vi "Initialization VI.vi"(8 "error in (no error)":errorcluster, 10 "Custom XML":string, 11 "Device Item Ref in":T1 format="%.0x") -> (0 "error out":errorcluster, 3 "Device Item Ref out":T1 format="%.0x")   [LabVIEW 2023, in "Vires VTD System Explorer.lvlib"]
uses:
  Vires VTD System Explorer.lvlib
  <vilib>/NI VeriStand/Custom Device API/Custom Device Item Ref.ctl
  Shared/Constants.vi
  <vilib>/NI VeriStand/Custom Device API/Custom Device API.lvlib
  Shared/Vires VTD Shared.lvlib
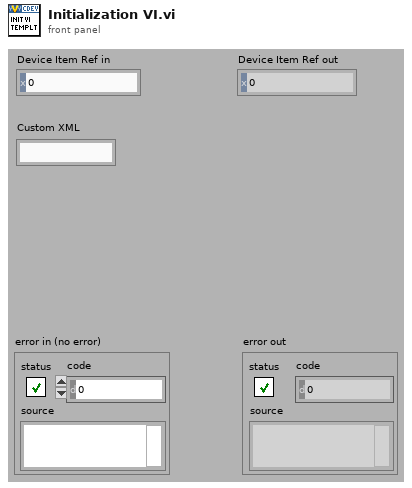
[diagram p1: front panel]
types:
  T1 = typedef "Custom Device API.lvlib/Custom Device Item Ref.ctl" = u64
  T2 = typedef "Vires VTD Shared.lvlib/Network Settings.ctl" = cluster{"IP adress":string, "RDB":cluster{"Protocol":T3, "Tx Port":u16, "Rx Port":u16, "Buffer Size":i32, "Timeout":u16}, "SCP":cluster{"Protocol":T3, "Tx Port":u16, "Rx Port":u16, "Buffer Size":i32, "Timeout":u16}}
  T3 = typedef "Vires VTD Shared.lvlib/Protocol.ctl" = enum16{"UDP", "TCP"}
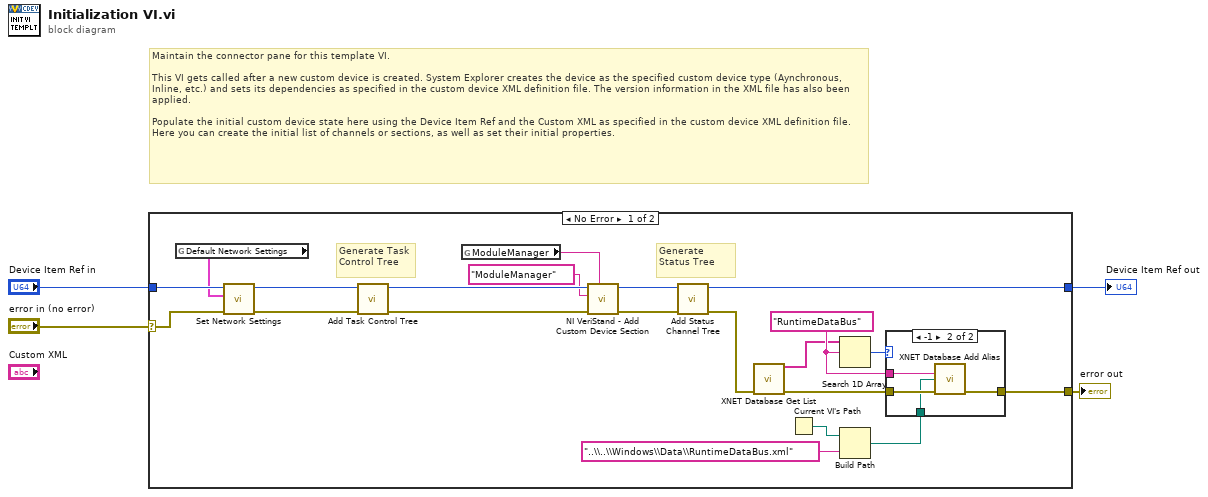
[diagram p0: block diagram]
diagram:
  # "Maintain the connector pane for this template VI.\n\nThis VI gets called after a new custom device is created. System Explorer creates the device as the specified custom device type (Aynchronous, Inline, etc.) and sets its dependencies as specified in the custom device XML definition file. The version information in the XML file has also been applied.\n\nPopulate the initial custom device state here using the Device Item Ref and the Custom XML as specified in the custom device XML definition file. Here you can create the initial list of channels or sections, as well as set their initial properties."
  n1 = case shown="No Error" "error in (no error)" {
    selector: "error in (no error)" -> [w13 w32]
    tunnel: [w17 w32] -> w1
    tunnel: [w19 w31] -> w3
    tunnel: "Device Item Ref in" -> [w15 w31]
    frame No Error {
      w23 = "RuntimeDataBus" ("element")
      # "Generate Status Tree"
      # "Generate Task Control Tree"
      n2 = global read "Constants.vi" "Default Network Settings"() -> (w9:T2)
      n3 = call "Set Network Settings.vi"("error in"=w13, "Network Settings"=w9, "Item Ref in"=w15) -> ("error out"=w12:errorcluster, "Item Ref out"=w14:T1)  [unwired: 7 in]
      n4 = call "Add Task Control Tree.vi"("error in (no error)"=w12, "Item Ref in"=w14) -> ("error out"=w11:errorcluster, "Parent Ref out"=w21:T1)  [unwired: 8 in]
      n5 = global read "Constants.vi" "ModuleManager"() -> (w22:string)
      n6 = call <vilib>:"NI VeriStand - Add Custom Device Section.vi"("GUID (Default Section)"=w22, "error in (no error)"=w11, "Section Name"="ModuleManager", "Parent Ref in"=w21) -> ("error out"=w18:errorcluster, "Parent Ref out"=w20:T1)  [unwired: 4 in, 2 out]
      n7 = call "Add Status Channel Tree.vi"("error in (no error)"=w18, "Parent Ref in"=w20) -> ("error out"=w16:errorcluster, "Parent Ref out"=w19:T1)  [unwired: 8 in]
      n8 = call <vilib>:"XNET Database Get List.vi"("error in (no error)"=w16) -> ("array of alias"=w8:string[], "error out"=w24:errorcluster)  [unwired: 12 in, 1 out]
      n9 = Current VI's Path() -> (path=w5:path)
      n10 = Search 1D Array(1D array=w8, element=w23) -> (index of element=w25:i32)  [unwired: 1 in]
      n11 = Build Path(base path=w5, name or relative path="..\\..\\Windows\\Data\\RuntimeDataBus.xml") -> (appended path=w6:path)
      n12 = case shown="-1" w25 {
        tunnel: w24 -> [w26 w30]
        tunnel: w23 -> [_ w29]
        tunnel: [w26 w28] -> w17
        tunnel: w6 -> [_ w27]
        frame 0, Default {
        }
        frame -1 {
          n13 = call <vilib>:"XNET Database Add Alias.vi"("alias"=w29, "filepath"=w27, "error in (no error)"=w30) -> ("error out"=w28:errorcluster)  [unwired: 12 in]
        }
      }
    }
    frame Error {
    }
  }
  "error out" <- w1
  "Device Item Ref out" <- w3
